vi "measureVPP.vi"(0 "OSC in":refnum<visa-resource-name>, 1 "error in (no error)":errorcluster) -> (2 "OSC out":refnum<visa-resource-name>, 3 "vpp":string, 4 "error out":errorcluster)   [LabVIEW 2016]
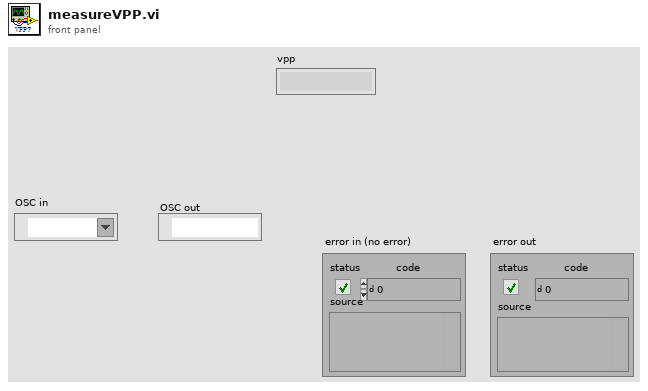
[diagram p1: front panel]
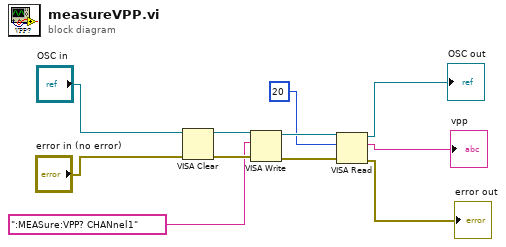
[diagram p0: block diagram]
diagram:
  n1 = VISA Clear(VISA resource name="OSC in", error in (no error)="error in (no error)") -> (VISA resource name out=w9:refnum<visa-resource-name>, error out=w8:errorcluster)
  n2 = VISA Write(VISA resource name=w9, write buffer=":MEASure:VPP? CHANnel1", error in (no error)=w8) -> (VISA resource name out=w6:refnum<visa-resource-name>, error out=w5:errorcluster)  [unwired: 1 out]
  n3 = VISA Read(VISA resource name=w6, byte count=20, error in (no error)=w5) -> (VISA resource name out=→"OSC out":refnum<visa-resource-name>, read buffer=→"vpp":string, error out=→"error out":errorcluster)  [unwired: 1 out]
